vi "Dequeue.vi"(6 "timeout in ms (-1)":i32=-1, 8 "error in (no error)":errorcluster, 11 "Message Queue":refnum<queue>) -> (0 "error out":errorcluster, 1 "Message Data":variant, 2 "State":T1=enum."Initialize", 3 "dup Message Queue":refnum<queue>, 4 "timed out?":bool, 5 "Call Chain":string[](array[string]))   [LabVIEW 2019, in "Message Queue.lvlib"]
doc: "This VI pulls messages off the Message Queue."
uses:
  Message Queue.lvlib
  Shared/TypeDefs/Message Queue Type.ctl
  State Name.ctl
  0f42f023-a962-4aed-ab19-c723e941f322.vi
  4f75f900-24ed-4a92-9154-8a6b05bc6094.vi
  <vilib>/Utility/error.llb/Clear Errors.vi
  <vilib>/Utility/error.llb/Error Cluster From Error Code.vi
panel:
  out "# elements in queue":i32
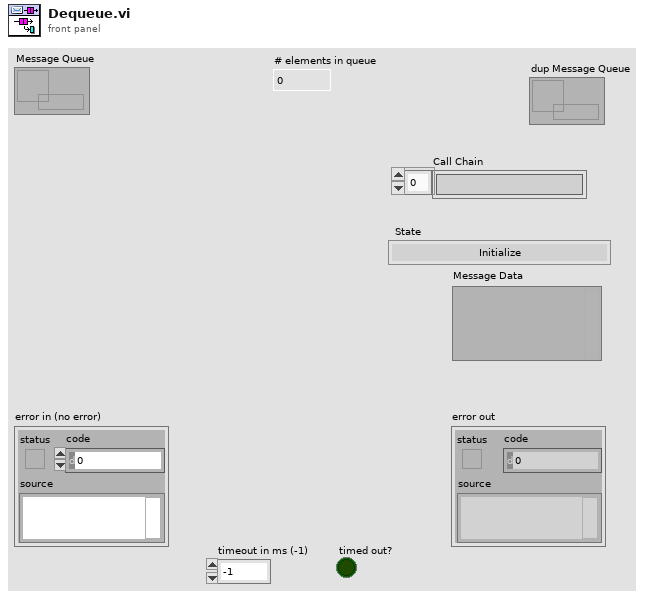
[diagram p1: front panel]
types:
  T1 = typedef "Message Queue.lvlib/State Name.ctl" = enum16{"Default", "Initialize", "Initialize Data", "Initialize Modules", "Initialize Panel", "Close FP", "Open FP", "Initialize Menu", "Mode", "Update Subpanel", "Error", "Open Help", "About", "Open WebResources", "Exit"}
  T2 = typedef "Message Queue Type.ctl" = cluster{"Custom State Name":string, "Defined State Name":variant, "Call Chain":string[], "Message Data":variant}
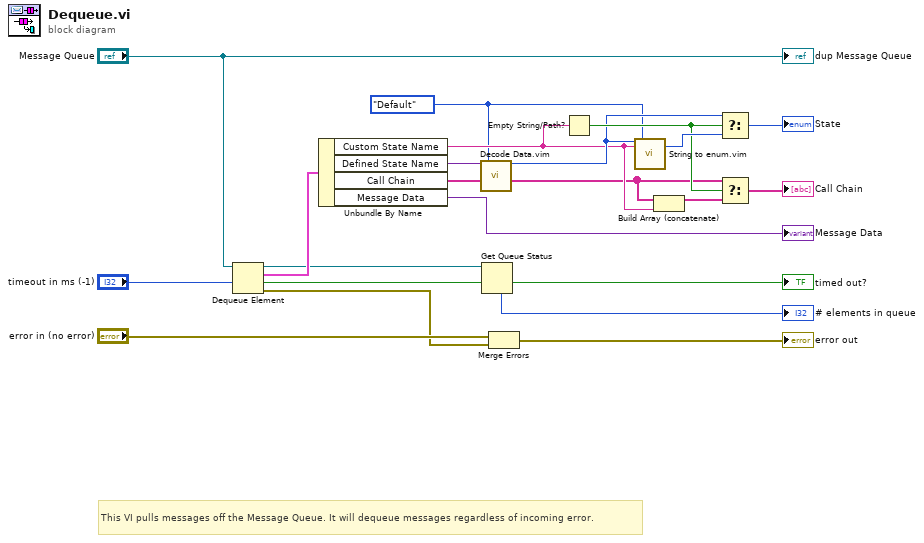
[diagram p0: block diagram]
diagram:
  w3 = State_Name."Default" ("State")
  # "This VI pulls messages off the Message Queue. It will dequeue messages regardless of incoming error."
  n1 = Dequeue Element(queue="Message Queue", timeout in ms (-1)="timeout in ms (-1)") -> (queue out=w15:refnum<queue>, element=w20:T2, timed out?=→"timed out?":bool, error out=w17:errorcluster)  [unwired: 1 in]
  n2 = Unbundle By Name(w20) -> ("Custom State Name"=w6:string, "Defined State Name"=w5:variant, "Call Chain"=w4:string[], "Message Data"=→"Message Data":variant)
  n3 = call "Decode Data.vim"("Data"=w5, "Type/Default value"=w3) -> ("Data out"=w7:T1)  [unwired: 16 in, 1 out]
  n4 = Get Queue Status(queue=w15) -> (# elements in queue=→"# elements in queue":i32)  [unwired: 2 in, 7 out]
  n5 = Merge Errors("error in (no error)", w17) -> (→"error out":errorcluster)
  n6 = Empty String/Path?(string/path=w6) -> (empty?=w9:bool)
  n7 = call "String to enum.vim"("Enum"=w7, "Item Name"=w6, "Default Item Name"=w3) -> ("Enum Selected"=w10:T1)  [unwired: 14 in, 2 out]
  n8 = Build Array (concatenate)(w4, w6) -> (w8:string[])
  n9 = Select(t=w7, s=w9, f=w10) -> (s? t:f=→"State":T1)
  n10 = Select(t=w4, s=w9, f=w8) -> (s? t:f=→"Call Chain":string[])
  "dup Message Queue" <- "Message Queue"
